vi "ForSoma.vi"() -> ()   [LabVIEW 2024]
panel:
  out "Meter":dbl(knob) scale=0.0..300.0
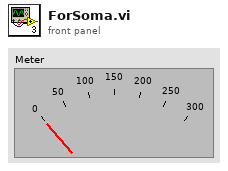
[diagram p1: front panel]
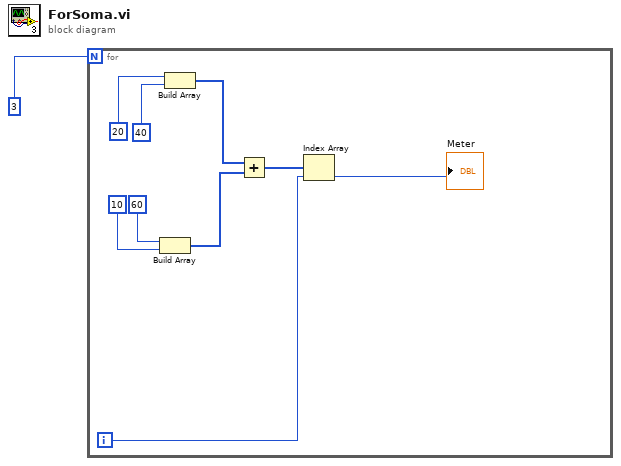
[diagram p0: block diagram]
diagram:
  n1 = for {
    N: 3 -> [_]
    i -> [w3]
    n2 = Build Array(60, 10) -> (w6:i32[])
    n3 = Build Array(20, 40) -> (w5:i32[])
    n4 = Add(x=w5, y=w6) -> (x+y=w4:i32[])
    n5 = Index Array(array=w4, index=w3) -> (element=→"Meter":i32)
  }
